vi "calcQx.vi"(5 "y2 Matrix":dbl[][](array[numeric]), 6 "Optical State":dbl[](array[numeric]), 7 "Weighting of Field Point":dbl[](array[numeric]), 8 "error in (no error)":errorcluster, 9 "Sen M":dbl[][][](array[numeric]), 10 "CC Matrix":dbl[][](array[numeric]), 11 "OptCtrl in":refnum<class "OptCtrl.lvclass">) -> (0 "error out":errorcluster, 2 "Qx Array":dbl[][](array[numeric]), 3 "OptCtrl out":refnum<class "OptCtrl.lvclass">)   [LabVIEW 2016, in "OfcFunc.lvlib" / "OptCtrl.lvclass"]
doc: "Calculate the Qx = sum_{wi * A.T * C.T * C * (A * yk+ y2k)}."
uses:
  OptCtrl.lvclass
  <vilib>/Analysis/baseanly.llb/Real A x B.vi
  <vilib>/Analysis/Matrix/Numeric/Conversions/Array To Matrix - RA2.vi
  <vilib>/Analysis/Matrix/Numeric/Add/Add - RM,RM.vi
  <vilib>/Analysis/Matrix/Numeric/Multiply/Multiply - R,RM.vi
  <vilib>/Analysis/Matrix/Numeric/Conversions/Matrix To Array - RM.vi
  <vilib>/Analysis/Matrix/NI_Matrix.lvlib
  <vilib>/Analysis/NI_AALBase.lvlib
  MatOper/MatOper.lvclass
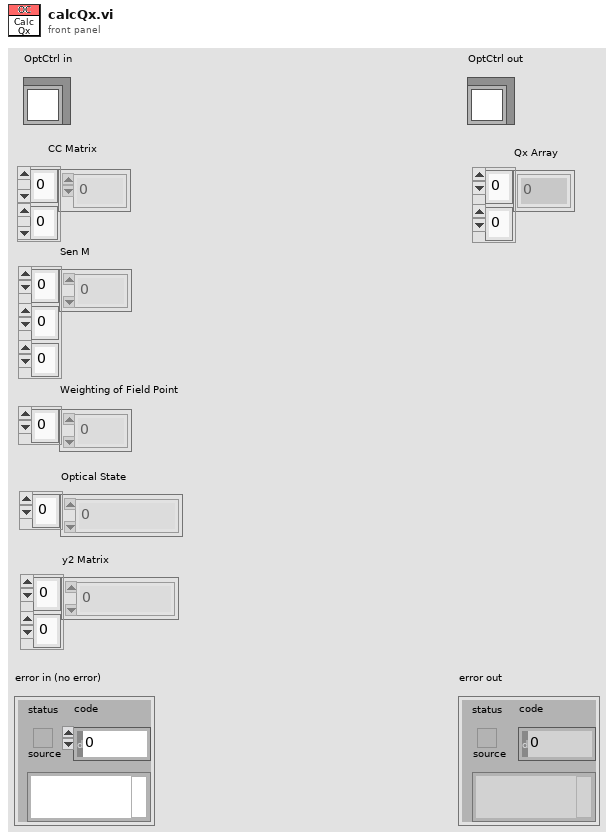
[diagram p1: front panel]
types:
  T1 = typedef "NI_Matrix.lvlib/RealMatrix.ctl" = dbl[][]
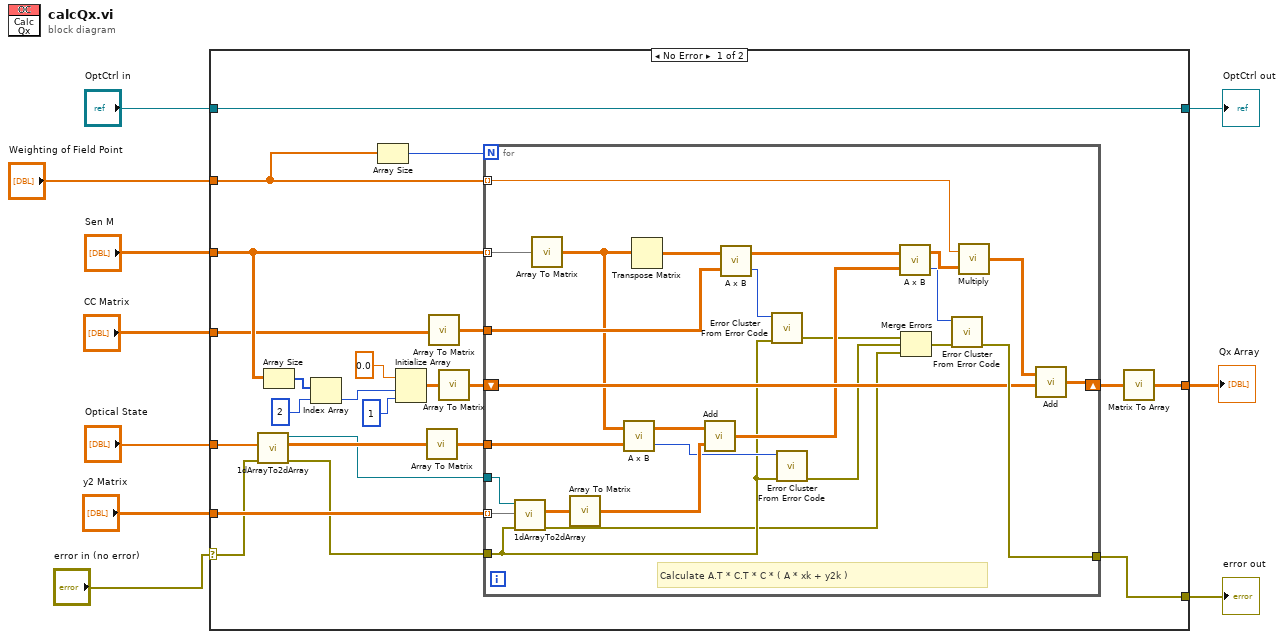
[diagram p0: block diagram]
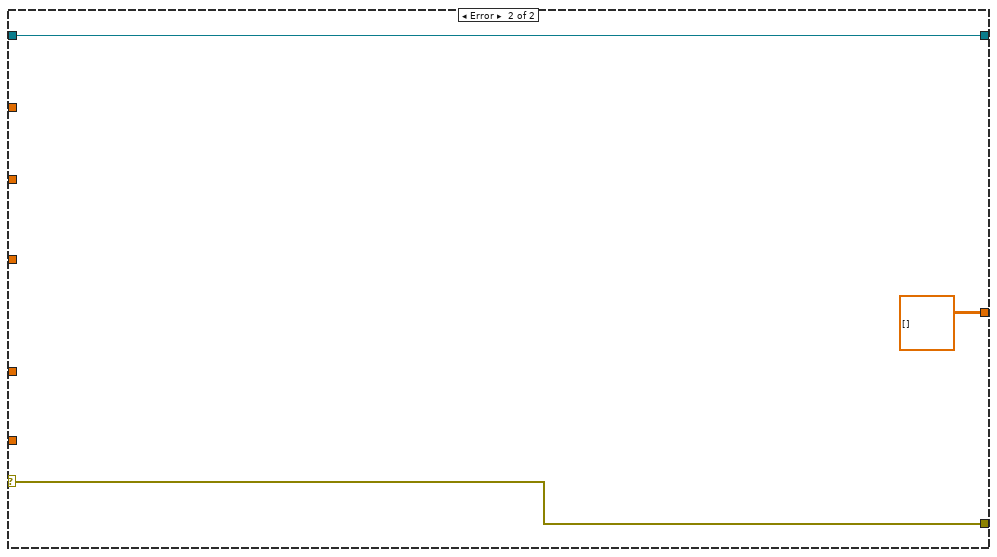
[diagram p2: hidden frame]
diagram:
  n1 = case shown="No Error" "error in (no error)" {
    selector: "error in (no error)" -> [w13 w62]
    tunnel: [w24 w62] -> w9
    tunnel: [w33 w61] -> w7
    tunnel: "OptCtrl in" -> [w33 w61]
    tunnel: "Weighting of Field Point" -> [w23 _]
    tunnel: "Sen M" -> [w22 _]
    tunnel: "CC Matrix" -> [w19 _]
    tunnel: "Optical State" -> [w21 _]
    tunnel: "y2 Matrix" -> [w16 _]
    tunnel: [w14 dbl[][] [] ("Real 2D Array")] -> w1
    frame No Error {
      n2 = call "1dArrayTo2dArray.vi"("error in (no error)"=w13, "1D Array"=w21) -> ("error out"=w12:errorcluster, "2D Array"=w18:dbl[][], "MatOper out"=w11:refnum<class "MatOper.lvclass">)  [unwired: 7 in]
      n3 = Array Size(array=w22) -> (size(s)=w29:i32[])
      n4 = Index Array(array=w29, index=2) -> (element=w27:i32)
      n5 = Array Size(array=w23) -> (size(s)=w31:i32)
      n6 = Initialize Array(0.0 ("element"), w27, 1 ("dimension size")) -> (w25:dbl[][])
      n7 = call-poly <vilib>:"Array To Matrix.vi"("Real 2D Array"=w18) -> ("Real Matrix"=w17:T1)
      n8 = call-poly <vilib>:"Array To Matrix.vi"("Real 2D Array"=w19) -> ("Real Matrix"=w20:T1)
      n9 = call-poly <vilib>:"Array To Matrix.vi"("Real 2D Array"=w25) -> ("Real Matrix"=w26:T1)
      n10 = for {
        N: w31 -> [_]
        tunnel: w23 -> [w56] mode=indexing
        tunnel: w22 -> [w59] mode=indexing
        shift-right: [w53] -> w32
        shift-left: w26 -> [w49]
        tunnel: w12 -> [w36]
        tunnel: [w50] -> w24
        tunnel: w20 -> [w48]
        tunnel: w17 -> [w44]
        tunnel: w16 -> [w47] mode=indexing
        tunnel: w11 -> [w34]
        # "Calculate A.T * C.T * C * ( A * xk + y2k )"
        n11 = call "1dArrayTo2dArray.vi"("error in (no error)"=w36, "1D Array"=w47, "MatOper in"=w34) -> ("error out"=w35:errorcluster, "2D Array"=w46:dbl[][])  [unwired: 6 in, 1 out]
        n12 = call-poly <vilib>:"Array To Matrix.vi"("Real 2D Array"=w59) -> ("Real Matrix"=w45:T1)
        n13 = call-poly <vilib>:"Array To Matrix.vi"("Real 2D Array"=w46) -> ("Real Matrix"=w42:T1)
        n14 = call-poly <vilib>:"A x B.vi"("B"=w44, "A"=w45) -> ("error"=w40:i32, "A x B"=w43:T1)
        n15 = Transpose Matrix(1:w45) -> (0:w58:T1)
        n16 = call-poly <vilib>:"Add.vi"("Real Matrix B"=w42, "Real Matrix A"=w43) -> ("A + B"=w41:T1)
        n17 = call-poly <vilib>:"A x B.vi"("B"=w48, "A"=w58) -> ("error"=w52:i32, "A x B"=w57:T1)
        n18 = call <vilib>:"Error Cluster From Error Code.vi"("error in (no error)"=w36, "error code (0)"=w52) -> ("error out"=w39:errorcluster)  [unwired: 7 in]
        n19 = call <vilib>:"Error Cluster From Error Code.vi"("error in (no error)"=w36, "error code (0)"=w40) -> ("error out"=w38:errorcluster)  [unwired: 7 in]
        n20 = call-poly <vilib>:"A x B.vi"("B"=w41, "A"=w57) -> ("error"=w51:i32, "A x B"=w55:T1)
        n21 = Merge Errors(w39, w38, w35) -> (w37:errorcluster)
        n22 = call <vilib>:"Error Cluster From Error Code.vi"("error in (no error)"=w37, "error code (0)"=w51) -> ("error out"=w50:errorcluster)  [unwired: 7 in]
        n23 = call-poly <vilib>:"Multiply.vi"("Real Matrix A"=w55, "Real Scalar c"=w56) -> ("c * A"=w54:T1)
        n24 = call-poly <vilib>:"Add.vi"("Real Matrix B"=w49, "Real Matrix A"=w54) -> ("A + B"=w53:T1)
      }
      n25 = call-poly <vilib>:"Matrix To Array.vi"("Real Matrix"=w32) -> ("Real 2D Array"=w14:dbl[][])
    }
    frame Error {
    }
  }
  "error out" <- w9
  "OptCtrl out" <- w7
  "Qx Array" <- w1
